vi "Run Action.vi"(8 "error in (no error)":errorcluster, 10 "Package":refnum<class "PackageAbstract.lvclass">, 11 "UpdateAction in":refnum<class "UpdateAction.lvclass">) -> (0 "error out":errorcluster, 2 "Problems":string[](array[string]), 3 "UpdateAction out":refnum<class "UpdateAction.lvclass">)   [LabVIEW 2020, in "GPackTools.lvlib" / "UpdateAction.lvclass"]
uses:
  UpdateAction.lvclass
  GPack/PackageAbstract/PackageAbstract.lvclass
  UpdateAction.lvclass/UpdateAction.ctl
  GPackTools.lvlib
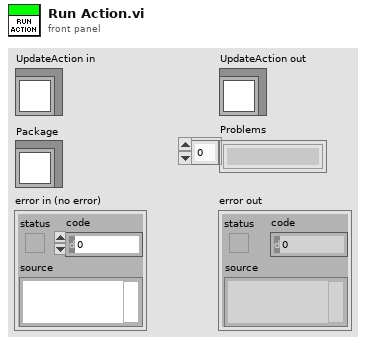
[diagram p1: front panel]
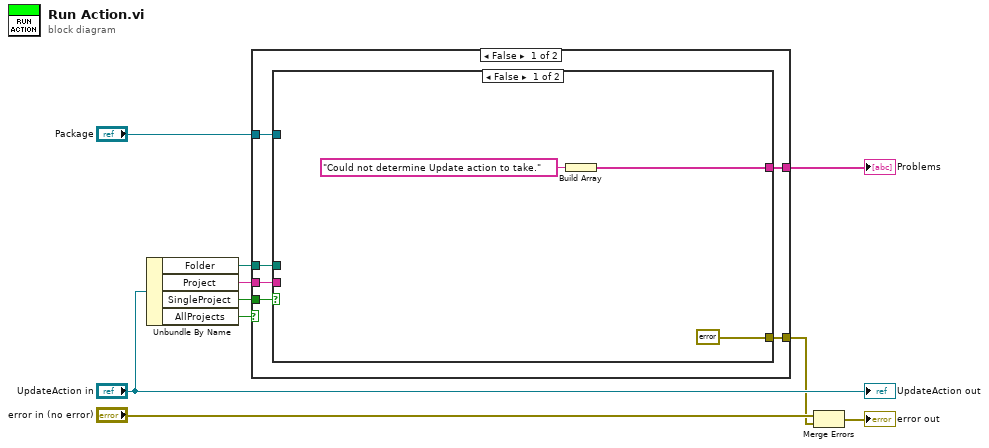
[diagram p0: block diagram]
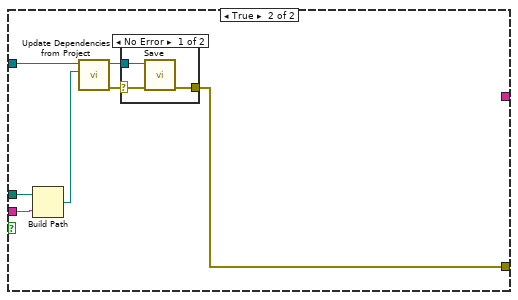
[diagram p2: hidden frame]
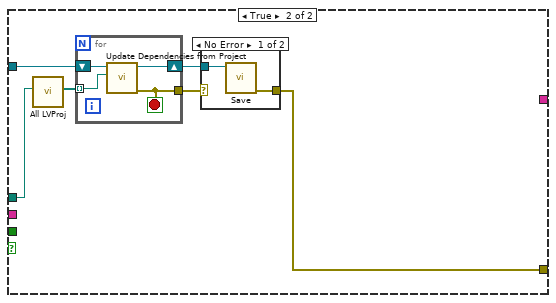
[diagram p4: hidden frame]
diagram:
  n1 = Unbundle By Name("UpdateAction in") -> ("Folder"=w4:path, "Project"=w6:string, "SingleProject"=w7:bool, "AllProjects"=w8:bool)
  n2 = case shown="False" w8 {
    tunnel: w7 -> [w16 _]
    tunnel: w6 -> [w15 _]
    tunnel: "Package" -> [w13 w35]
    tunnel: w4 -> [w14 w36]
    tunnel: [w12 w31] -> w2
    tunnel: [w11 _] -> w1
    frame False {
      n3 = case shown="False" w16 {
        tunnel: w15 -> [_ w25]
        tunnel: w14 -> [_ w26]
        tunnel: w13 -> [_ w24]
        tunnel: [errorcluster {"status"=FALSE, "code"=0, "source"=""} ("error IO") w20] -> w12
        tunnel: [w17 _] -> w11
        frame False {
          n4 = Build Array("Could not determine Update action to take.") -> (w17:string[])
        }
        frame True {
          n5 = Build Path(base path=w26, name or relative path=w25) -> (appended path=w23:path)
          n6 = call "Update Dependencies from Project.vi"("lvproj Path"=w23, "PackageAbstract in"=w24) -> ("error out"=w22:errorcluster, "PackageAbstract out"=w21:refnum<class "PackageAbstract.lvclass">)  [unwired: 8 in]
          n7 = case shown="No Error" w22 {
            selector: w22 -> [w28 w30]
            tunnel: w21 -> [w29 _]
            tunnel: [w27 w30] -> w20
            frame No Error {
              n8 = call "Save.vi"("error in (no error)"=w28, "PackageAbstract in"=w29) -> ("error out"=w27:errorcluster)  [unwired: 8 in, 1 out]
            }
            frame Error {
            }
          }
        }
      }
    }
    frame True {
      n9 = call "All LVProj.vi"("Folder"=w36) -> ("All LVProj"=w34:path[])  [unwired: 10 in]
      n10 = for {
        shift-right: [w42] -> w32
        shift-left: w35 -> [w43]
        tunnel: w34 -> [w41] mode=indexing
        tunnel: [w40] -> w33
        stop <- w40 stop-if-true
        n11 = call "Update Dependencies from Project.vi"("lvproj Path"=w41, "PackageAbstract in"=w43) -> ("error out"=w40:errorcluster, "PackageAbstract out"=w42:refnum<class "PackageAbstract.lvclass">)  [unwired: 8 in]
      }
      n12 = case shown="No Error" w33 {
        selector: w33 -> [_ w39]
        tunnel: w32 -> [w38 _]
        tunnel: [w37 w39] -> w31
        frame No Error {
          n13 = call "Save.vi"("PackageAbstract in"=w38) -> ("error out"=w37:errorcluster)  [unwired: 9 in, 1 out]
        }
        frame Error {
        }
      }
    }
  }
  "Problems" <- w1
  n14 = Merge Errors("error in (no error)", w2) -> (→"error out":errorcluster)
  "UpdateAction out" <- "UpdateAction in"
